vi "SP Read.vi"   [LabVIEW 2023, in "Setpoint.lvclass"]
uses:
  Setpoint.lvclass
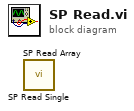
[diagram p0: block diagram]
diagram:
  n1 = call "SP Read Single.vi"() -> ()  [unwired: 8 in, 4 out]
  n2 = call "SP Read Array.vi"() -> ()  [unwired: 8 in, 4 out]
